vi "StreamTransmitAcquisitionChA.vi"() -> ()   [LabVIEW 2018]
uses:
  <resource>/objmgr/ni.dex.rc
panel:
  in  "stop 3":bool
  out "error out 4":errorcluster
  in  "Cluster":cluster{"Address":string, "Remote Port":u32}
  in  "stop 2":bool
  out "error out 3":errorcluster
  out "error out 2":errorcluster
  out "error out":errorcluster
  in  "stop":bool
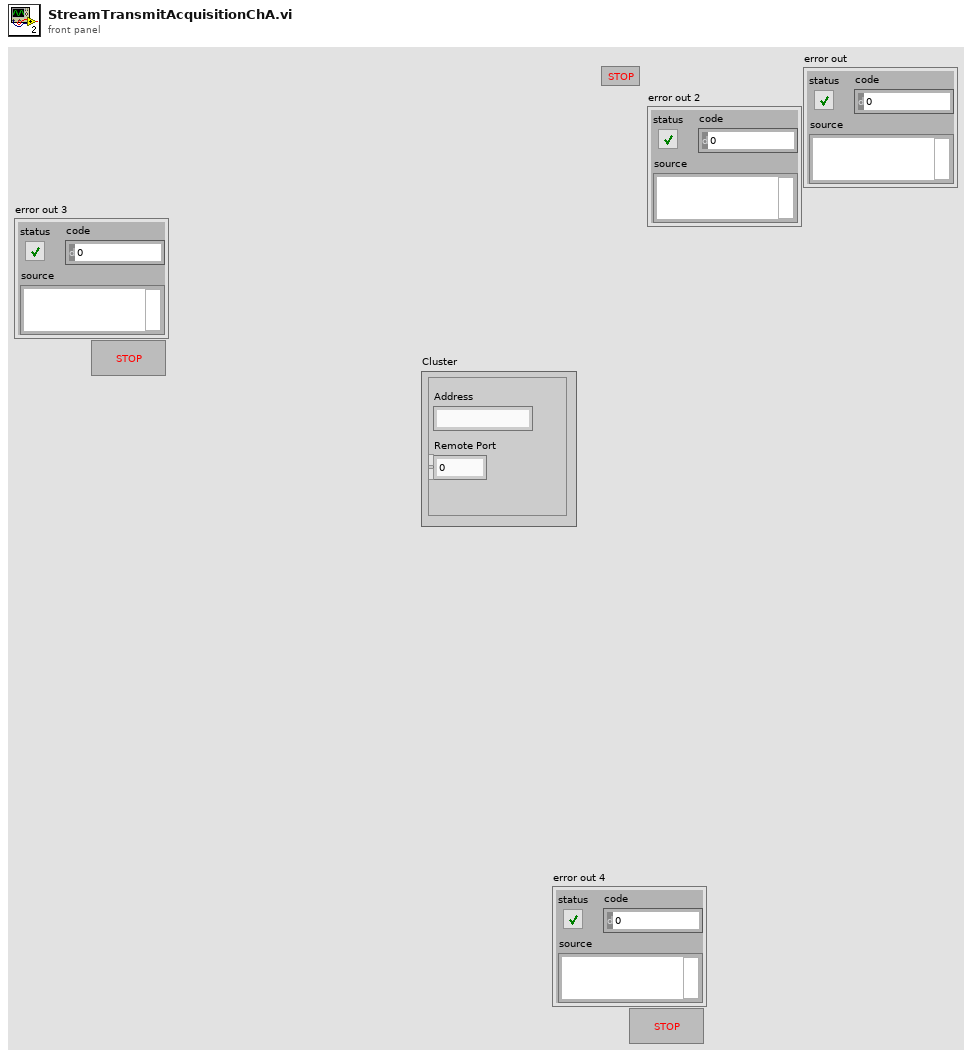
[diagram p1: front panel]
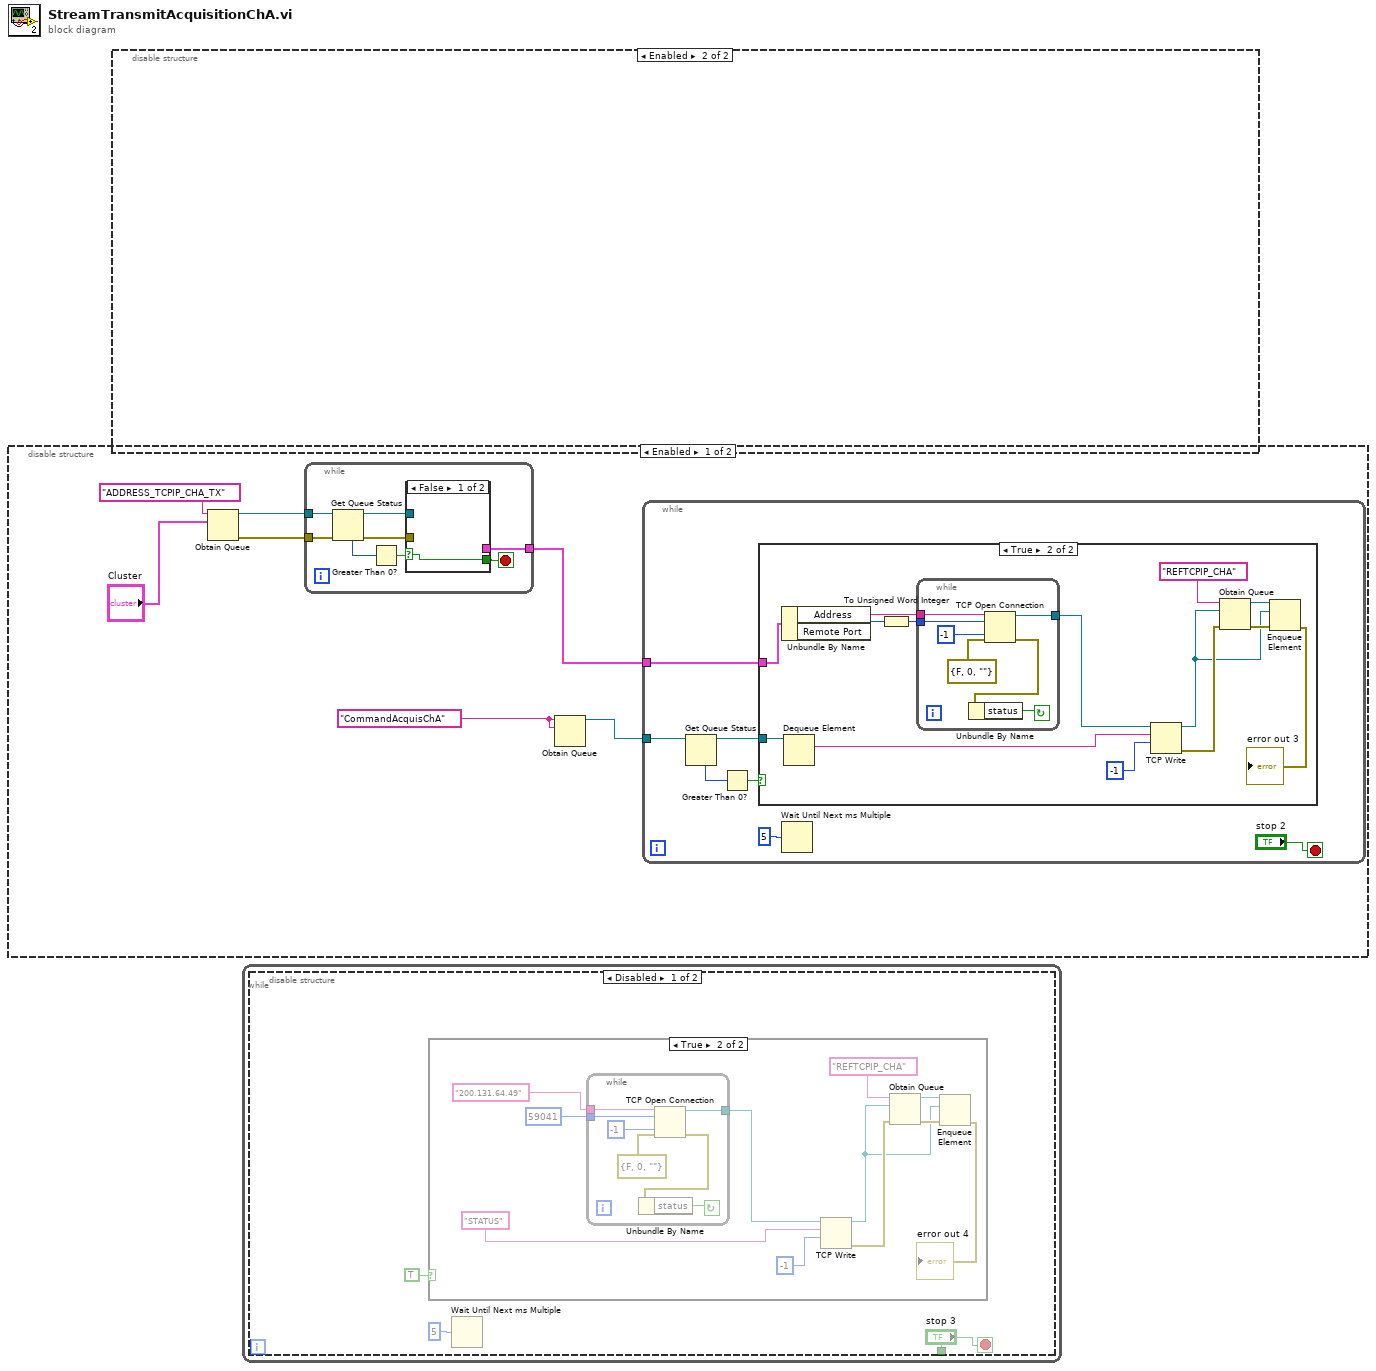
[diagram p0: block diagram]
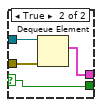
[diagram p2: hidden frame]
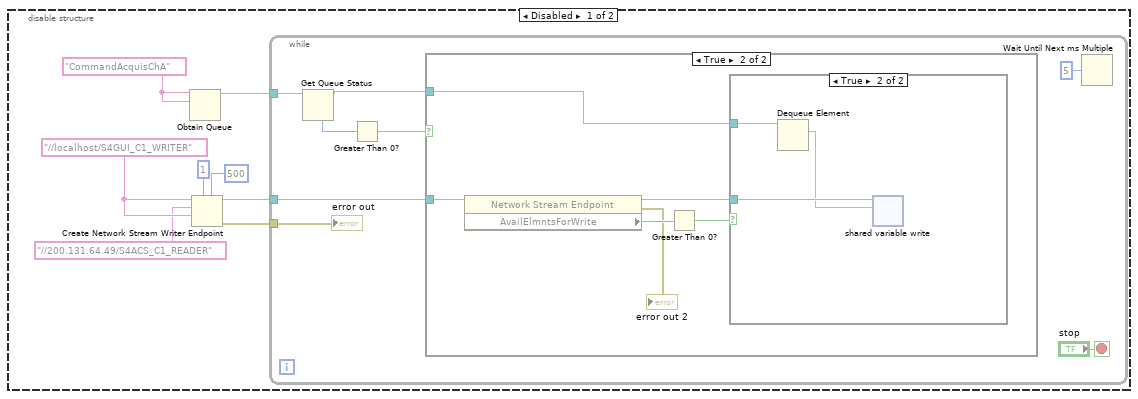
[diagram p7: hidden frame]
diagram:
  n1 = disable-structure shown="Enabled" {
    frame Enabled {
      w1 = "CommandAcquisChA"
      n2 = Obtain Queue(name (unnamed)="ADDRESS_TCPIP_CHA_TX", element data type="Cluster") -> (queue out=w3:refnum<queue>, error out=w4:errorcluster)  [unwired: 3 in, 1 out]
      n3 = while {
        tunnel: [w15] -> w5
        tunnel: w4 -> [w13]
        tunnel: w3 -> [w12]
        stop <- w8 stop-if-true
        n4 = Get Queue Status(queue=w12, error in (no error)=w13) -> (queue out=w11:refnum<queue>, error out=w14:errorcluster, # elements in queue=w10:i32)  [unwired: 1 in, 5 out]
        n5 = Greater Than 0?(x=w10) -> (x > 0?=w9:bool)
        n6 = case shown="False" w9 {
          selector: w9 -> [w16 w17]
          tunnel: [_ w20] -> w15
          tunnel: w14 -> [_ w19]
          tunnel: w11 -> [_ w18]
          tunnel: [w16 w17] -> w8
          frame False {
          }
          frame True {
            n7 = Dequeue Element(queue=w18, error in (no error)=w19) -> (element=w20:cluster{"Address":string, "Remote Port":u32})  [unwired: 1 in, 3 out]
          }
        }
      }
      n8 = Obtain Queue(name (unnamed)=w1, element data type=w1) -> (queue out=w7:refnum<queue>)  [unwired: 3 in, 2 out]
      n9 = while {
        tunnel: w7 -> [w26]
        tunnel: w5 -> [w21]
        stop <- "stop 2" stop-if-true
        n10 = Get Queue Status(queue=w26) -> (queue out=w23:refnum<queue>, # elements in queue=w25:i32)  [unwired: 2 in, 6 out]
        n11 = Greater Than 0?(x=w25) -> (x > 0?=w24:bool)
        n12 = case shown="True" w24 {
          tunnel: w23 -> [_ w41]
          tunnel: w21 -> [_ w39]
          frame False {
          }
          frame True {
            n13 = Unbundle By Name(w39) -> ("Address"=w29:string, "Remote Port"=w28:u32)
            n14 = Dequeue Element(queue=w41) -> (element=w40:string)  [unwired: 2 in, 3 out]
            n15 = To Unsigned Word Integer(number=w28) -> (unsigned 16bit integer=w30:u16)
            n16 = while {
              tunnel: [w48] -> w38
              tunnel: w30 -> [w47]
              tunnel: w29 -> [w46]
              stop <- w42 continue-if-true
              n17 = TCP Open Connection(address=w46, remote port or service name=w47, timeout ms (60000)=-1, error in (no error)=errorcluster {"status"=FALSE, "code"=0, "source"=""}) -> (connection ID=w48:refnum<k5>, error out=w43:errorcluster)  [unwired: 1 in]
              n18 = Unbundle By Name(w43) -> ("status"=w42:bool)
            }
            n19 = TCP Write(connection ID=w38, data in=w40, 9:-1 ("timeout ms (25000)")) -> (connection ID out=w34:refnum<k5>, error out=w36:errorcluster)  [unwired: 1 in, 1 out]
            n20 = Obtain Queue(name (unnamed)="REFTCPIP_CHA", element data type=w34, error in (no error)=w36) -> (queue out=w33:refnum<queue>, error out=w35:errorcluster)  [unwired: 2 in, 1 out]
            n21 = Enqueue Element(queue=w33, element=w34, error in (no error)=w35) -> (error out=→"error out 3":errorcluster)  [unwired: 1 in, 2 out]
          }
        }
        n22 = Wait Until Next ms Multiple(millisecond multiple=u32 5) -> ()  [unwired: 1 out]
      }
    }
    frame Disabled {
    }
  }
  n23 = disable-structure shown="Enabled" {
    frame Disabled {
      w52 = "//localhost/S4GUI_C1_WRITER"
      w53 = "CommandAcquisChA"
      n24 = Obtain Queue(name (unnamed)=w53, element data type=w53) -> (queue out=w56:refnum<queue>)  [unwired: 3 in, 2 out]
      n25 = Create Network Stream Writer Endpoint(5:500 ("timeout in ms (-1)"), 7:1 ("writer buffer size"), 9:w52, 10:"//200.131.64.49/S4ACS_C1_READER", 11:w52) -> (0:w49:errorcluster, 3:w54:refnum<k21>)  [unwired: 2 in]
      n26 = while {
        tunnel: w56 -> [w63]
        tunnel: w54 -> [w59]
        tunnel: w49 -> [w57]
        stop <- "stop" stop-if-true
        n27 = Get Queue Status(queue=w63) -> (queue out=w60:refnum<queue>, # elements in queue=w62:i32)  [unwired: 2 in, 6 out]
        n28 = Greater Than 0?(x=w62) -> (x > 0?=w61:bool)
        n29 = case shown="True" w61 {
          tunnel: w60 -> [_ w70]
          tunnel: w59 -> [_ w69]
          frame False {
          }
          frame True {
            n30 = property class="Network Stream Endpoint"(reference=w69) -> (reference out=w66:refnum<k21>, error out=→"error out 2":errorcluster, "AvailElmntsForWrite"=w68:i32)  [unwired: 1 in]
            n31 = Greater Than 0?(x=w68) -> (x > 0?=w67:bool)
            n32 = case shown="True" w67 {
              tunnel: w70 -> [_ w73]
              tunnel: w66 -> [_ w72]
              frame False {
              }
              frame True {
                n33 = Dequeue Element(queue=w73) -> (element=w71:string)  [unwired: 2 in, 3 out]
                n34 = shared-variable-write(w72, w71) -> ()  [unwired: 2 in, 3 out]
              }
            }
          }
        }
        n35 = Wait Until Next ms Multiple(millisecond multiple=u32 5) -> ()  [unwired: 1 out]
        "error out" <- w57
      }
    }
    frame Enabled {
    }
  }
  n36 = while {
    stop <- w74 stop-if-true
    n37 = disable-structure shown="Disabled" {
      disable-tunnel: ["stop 3" _] -> w74
      frame Disabled {
        n38 = case shown="True" TRUE {
          frame False {
          }
          frame True {
            n39 = while {
              tunnel: [w95] -> w88
              tunnel: u16 59041 -> [w94]
              tunnel: "200.131.64.49" -> [w93]
              stop <- w89 continue-if-true
              n40 = TCP Open Connection(address=w93, remote port or service name=w94, timeout ms (60000)=-1, error in (no error)=errorcluster {"status"=FALSE, "code"=0, "source"=""}) -> (connection ID=w95:refnum<k5>, error out=w90:errorcluster)  [unwired: 1 in]
              n41 = Unbundle By Name(w90) -> ("status"=w89:bool)
            }
            n42 = TCP Write(connection ID=w88, data in="STATUS", 9:-1 ("timeout ms (25000)")) -> (connection ID out=w84:refnum<k5>, error out=w86:errorcluster)  [unwired: 1 in, 1 out]
            n43 = Obtain Queue(name (unnamed)="REFTCPIP_CHA", element data type=w84, error in (no error)=w86) -> (queue out=w83:refnum<queue>, error out=w85:errorcluster)  [unwired: 2 in, 1 out]
            n44 = Enqueue Element(queue=w83, element=w84, error in (no error)=w85) -> (error out=→"error out 4":errorcluster)  [unwired: 1 in, 2 out]
          }
        }
        n45 = Wait Until Next ms Multiple(millisecond multiple=u32 5) -> ()  [unwired: 1 out]
      }
      frame Enabled {
      }
    }
  }
